vi "getFuncReturn.vi"(8 "error in (no error)":errorcluster, 10 "referenceIn":refnum<vi>, 11 "SalProcess in":refnum<class "SalProcess.lvclass">) -> (0 "error out":errorcluster, 1 "function return":i32, 2 "referenceOut":refnum<vi>, 3 "SalProcess out":refnum<class "SalProcess.lvclass">)   [LabVIEW 2018, in "SalProcess.lvclass"]
doc: "Get the SAL function return."
uses:
  SalProcess.lvclass
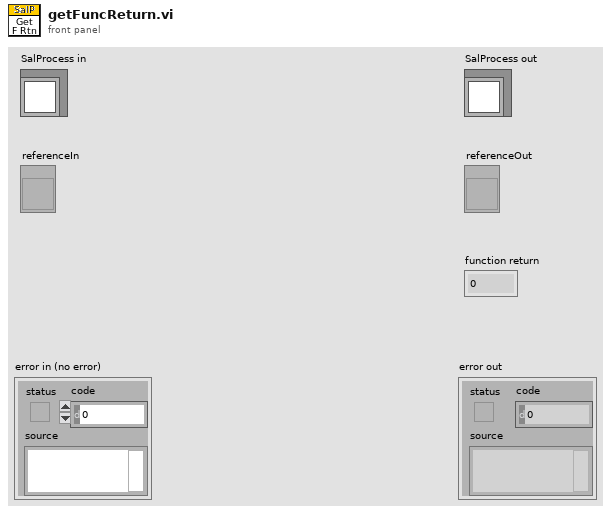
[diagram p1: front panel]
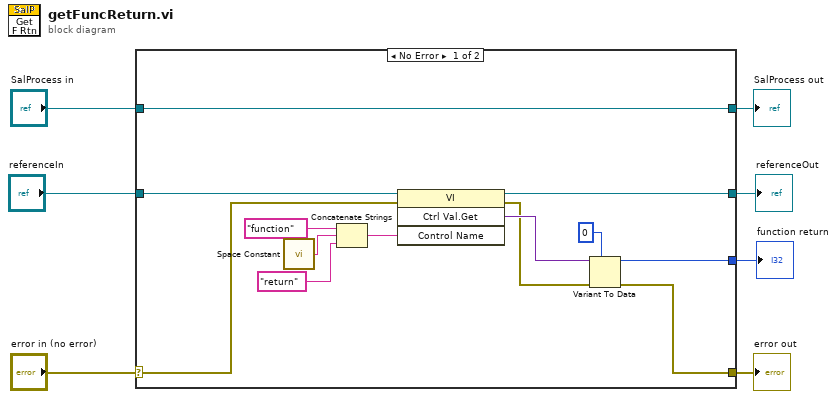
[diagram p0: block diagram]
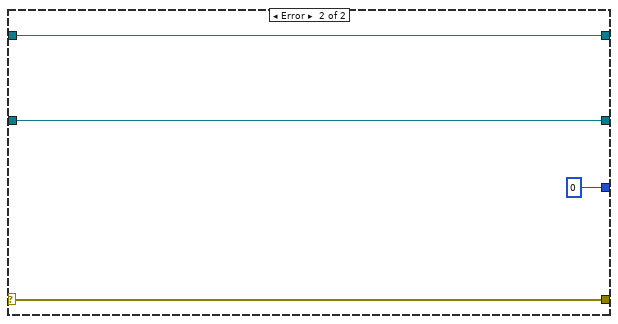
[diagram p2: hidden frame]
diagram:
  n1 = case shown="No Error" "error in (no error)" {
    selector: "error in (no error)" -> [w10 w24]
    tunnel: [w11 w24] -> w6
    tunnel: [w20 w23] -> w4
    tunnel: "SalProcess in" -> [w20 w23]
    tunnel: [w12 0] -> w3
    tunnel: [w9 w21] -> w1
    tunnel: "referenceIn" -> [w8 w21]
    frame No Error {
      n2 = call <vilib>:"Space Constant.vi"() -> ("String"=w18:string)
      n3 = Concatenate Strings("function", w18, "return") -> (w16:string)
      n4 = invoke class="VI" method="Ctrl Val.Get"(reference=w8, error in=w10, "Control Name"=w16) -> (reference out=w9:refnum<vi>, error out=w13:errorcluster, "Get Control Value Variant"=w15:variant)  [unwired: 1 in, 1 out]
      n5 = Variant To Data(error in=w13, type=0, Variant=w15) -> (data=w12:i32, error out=w11:errorcluster)
    }
    frame Error {
    }
  }
  "error out" <- w6
  "SalProcess out" <- w4
  "function return" <- w3
  "referenceOut" <- w1
